vi "frequency_analysis.vi"(7 "Analizza":bool, 8 "data":waveform(dbl)[](array[waveform]), 9 "Fgen freq":dbl, 10 "XY Phase in":cluster{dbl[], dbl[]}[](array[cluster]), 11 "XY Amp in":cluster{dbl[], dbl[]}[](array[cluster])) -> (2 "XY Phase out":cluster{dbl[], dbl[]}[](array[cluster]), 3 "XY Amp out":cluster{dbl[], dbl[]}[](array[cluster]))   [LabVIEW 2023]
uses:
  <vilib>/measure/matone.llb/Extract Single Tone Information 1 Chan.vi
  <vilib>/gmath/NumericalOptimization/Nonlinear Curve Fit LM.vi
  <vilib>/measure/NI_MAPro.lvlib
  <vilib>/gmath/NI_Gmath.lvlib
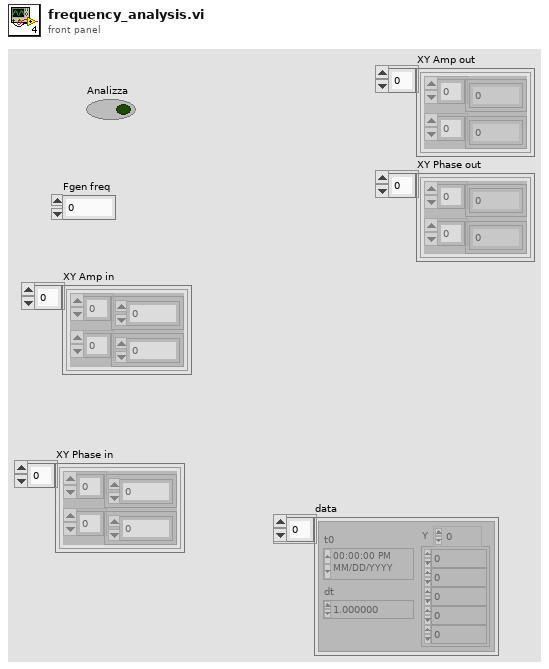
[diagram p1: front panel]
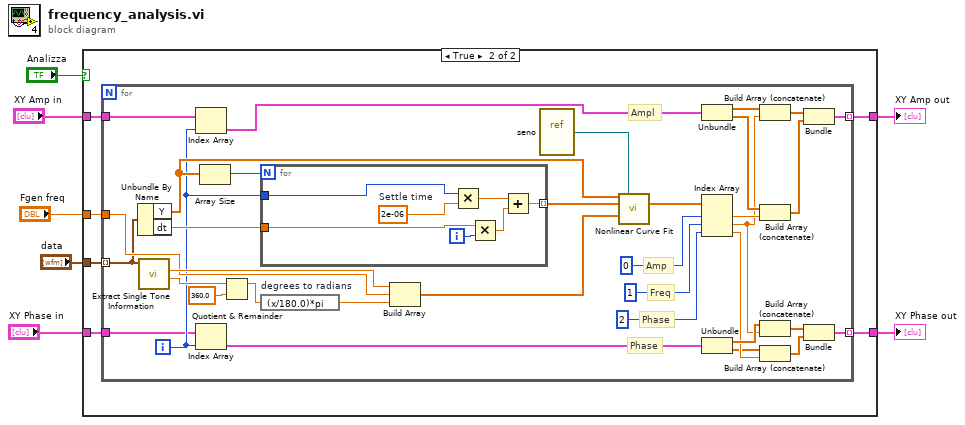
[diagram p0: block diagram]
diagram:
  n1 = case shown="True" "Analizza" {
    tunnel: "data" -> [_ w15]
    tunnel: "Fgen freq" -> [_ w14]
    tunnel: [w9 w13] -> w5
    tunnel: [w8 w12] -> w4
    tunnel: "XY Amp in" -> [w9 w11]
    tunnel: "XY Phase in" -> [w8 w10]
    frame False {
    }
    frame True {
      n2 = for {
        tunnel: w15 -> [w42] mode=indexing
        tunnel: w14 -> [w44]
        tunnel: [w26] -> w13 mode=indexing
        tunnel: [w25] -> w12 mode=indexing
        tunnel: w11 -> [w20]
        tunnel: w10 -> [w17]
        i -> [w18]
        # "Phase"
        # "Ampl"
        # "Phase"
        # "Freq"
        # "Amp"
        n3 = Unbundle By Name(w42) -> ("Y"=w49:dbl[], "dt"=w47:dbl)
        n4 = call-poly <vilib>:"Extract Single Tone Information.vi"("time signal in"=w42) -> ("detected phase (deg)"=w23:dbl, "detected amplitude"=w45:dbl)  [unwired: 5 in, 4 out]
        n5 = Index Array(array=w20, index=w18) -> (element=w19:cluster{dbl[], dbl[]})
        n6 = Index Array(array=w17, index=w18) -> (element=w16:cluster{dbl[], dbl[]})
        n7 = Array Size(array=w49) -> (size(s)=w48:i32)
        n8 = Quotient & Remainder(x=w23, y=360.0) -> (x-y*floor(x/y)=w21:dbl)  [unwired: 1 out]
        n9 = for {
          N: w48 -> [_]
          tunnel: w47 -> [w56]
          tunnel: [w55] -> w46 mode=indexing
          tunnel: w18 -> [w53]
          i -> [w57]
          w52 = 2e-06  # Settle time
          n10 = Multiply(x=w53, y=w52) -> (x*y=w51:dbl)
          n11 = Multiply(x=w56, y=w57) -> (x*y=w54:dbl)
          n12 = Add(x=w51, y=w54) -> (x+y=w55:dbl)
        }
        n13 = expression code="(x/180.0)*pi" "degrees to radians"(w21) -> (w24:dbl)
        n14 = Build Array(w45, w44, w24) -> (w43:dbl[])
        n15 = vi-ref "seno.vi"() -> (w50:refnum<vi>)
        n16 = call-poly <vilib>:"Nonlinear Curve Fit.vi"("Y"=w49, "f(x,a)"=w50, "X"=w46, "initial parameters"=w43) -> ("best fit parameters"=w41:dbl[])  [unwired: 6 in, 5 out]
        n17 = Unbundle(w19) -> (w37:dbl[], w36:dbl[])
        n18 = Index Array(array=w41, index #1=0 ("index"), index #2=1 ("index"), index #3=2 ("index")) -> (element #1=w35:dbl, element #2=w33:dbl, element #3=w32:dbl)
        n19 = Unbundle(w16) -> (w34:dbl[], w31:dbl[])
        n20 = Build Array (concatenate)(w37, w33) -> (w30:dbl[])
        n21 = Build Array (concatenate)(w36, w35) -> (w29:dbl[])
        n22 = Build Array (concatenate)(w34, w33) -> (w28:dbl[])
        n23 = Build Array (concatenate)(w31, w32) -> (w27:dbl[])
        n24 = Bundle(w30, w29) -> (w26:cluster{dbl[], dbl[]})  [unwired: 1 in]
        n25 = Bundle(w28, w27) -> (w25:cluster{dbl[], dbl[]})  [unwired: 1 in]
      }
    }
  }
  "XY Amp out" <- w5
  "XY Phase out" <- w4
